vi "add channel.vi"(6 "replace if found?(T)":bool, 8 "error in (no error)":errorcluster, 9 "DSFChannel info":T1, 10 "id":string, 11 "DSFConfiguration in":refnum<class "DSFConfiguration.lvclass">) -> (0 "error out":errorcluster, 1 "found?":bool, 3 "DSFConfiguration out":refnum<class "DSFConfiguration.lvclass">)   [LabVIEW 2017, in "DSFConfiguration.lvclass"]
uses:
  DSFConfiguration.lvclass
  DSFConfiguration.lvclass/DSFConfiguration.ctl
  DSFChannel/DSFChannel.lvclass
  <vilib>/Utility/error.llb/Error Cluster From Error Code.vi
  <vilib>/ErrorRing/Error Ring.xnode
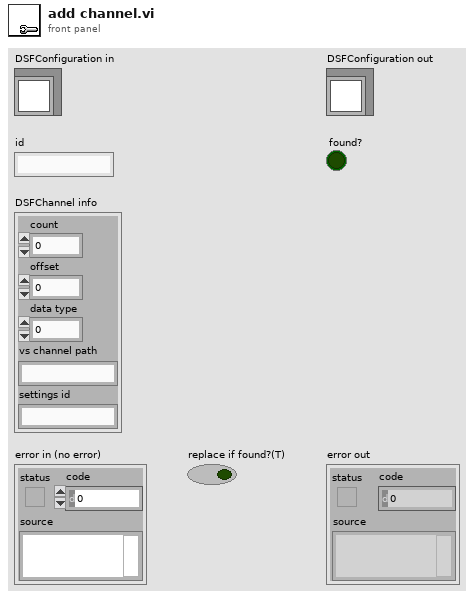
[diagram p1: front panel]
types:
  T1 = cluster{"count":i32, "offset":i32, "data type":i32, "vs channel path":string, "settings id":string}
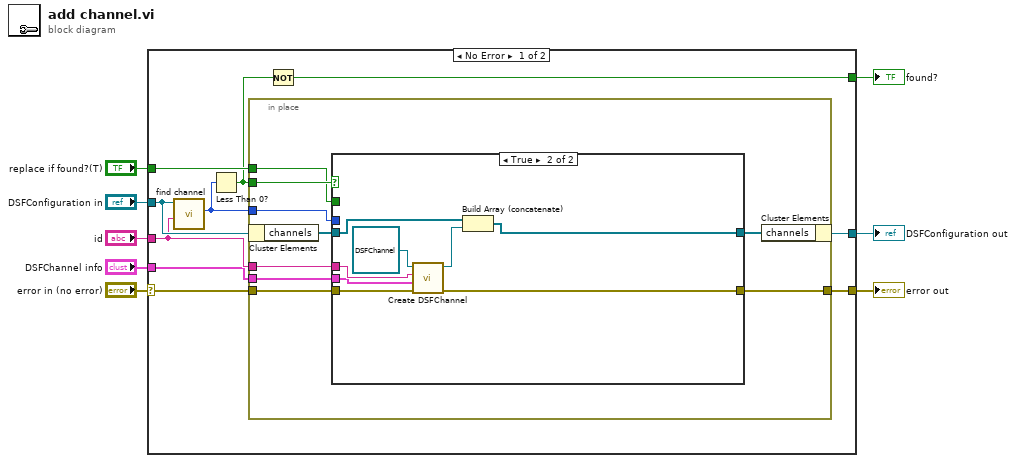
[diagram p0: block diagram]
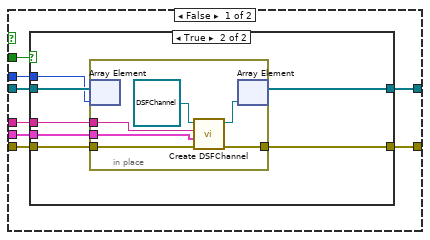
[diagram p2: hidden frame]
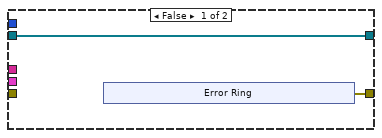
[diagram p3: hidden frame]
diagram:
  n1 = case shown="No Error" "error in (no error)" {
    selector: "error in (no error)" -> [w13 w64]
    tunnel: [w12 w64] -> w7
    tunnel: [w15 w63] -> w5
    tunnel: "DSFConfiguration in" -> [w18 w63]
    tunnel: "replace if found?(T)" -> [w17 _]
    tunnel: "id" -> [w14 _]
    tunnel: [w10 _] -> w2
    tunnel: "DSFChannel info" -> [w9 _]
    frame No Error {
      n2 = call "find channel.vi"("settings id"=w14, "DSFConfiguration in"=w18) -> ("index"=w16:i32)  [unwired: 9 in]
      n3 = Less Than 0?(x=w16) -> (x < 0?=w11:bool)
      n4 = in-place {
        in-place-border: w11 -> [w26]
        in-place-border: w14 -> [w25]
        in-place-border: w17 -> [w24]
        in-place-border: w16 -> [w23]
        in-place-border: w13 -> [w22]
        in-place-border: [w21] -> w12
        in-place-border: w9 -> [w20]
        n5 = in-place-cluster #1(w18) -> ("channels"=w27:refnum<class "DSFChannel.lvclass">[])
        n6 = case shown="True" w26 {
          tunnel: w27 -> [w35 w62]
          tunnel: w25 -> [w32 w59]
          tunnel: [w31 w61] -> w19
          tunnel: w24 -> [w34 _]
          tunnel: w23 -> [w33 _]
          tunnel: w22 -> [w30 w58]
          tunnel: [w29 w56] -> w21
          tunnel: w20 -> [w28 w55]
          frame False {
            n7 = case shown="True" w34 {
              tunnel: w35 -> [w37 w48]
              tunnel: w33 -> [_ w47]
              tunnel: w32 -> [_ w46]
              tunnel: [w37 w45] -> w31
              tunnel: w30 -> [_ w44]
              tunnel: [w36 w43] -> w29
              tunnel: w28 -> [_ w42]
              frame False {
                n8 = xnode "Error Ring"() -> ("error out"=w36:errorcluster)
              }
              frame True {
                n9 = in-place {
                  in-place-border: w46 -> [w53]
                  in-place-border: w44 -> [w51]
                  in-place-border: [w50] -> w43
                  in-place-border: w42 -> [w49]
                  n10 = in-place-array #2(w48, w47) -> ()  [unwired: 1 out]
                  n11 = call "Create DSFChannel.vi"("error in (no error)"=w51, "DSFChannel info"=w49, "id"=w53, "DSFChannel in"=refnum<class "DSFChannel.lvclass"> refnum ("DSFPluginSettings in")) -> ("error out"=w50:errorcluster, "DSFChannel out"=w52:refnum<class "DSFChannel.lvclass">)  [unwired: 6 in]
                  n12 = in-place-array #2(w52) -> (w45:refnum<class "DSFChannel.lvclass">[])  [unwired: 1 out]
                }
              }
            }
          }
          frame True {
            n13 = call "Create DSFChannel.vi"("error in (no error)"=w58, "DSFChannel info"=w55, "id"=w59, "DSFChannel in"=refnum<class "DSFChannel.lvclass"> refnum ("DSFPluginSettings in")) -> ("error out"=w56:errorcluster, "DSFChannel out"=w57:refnum<class "DSFChannel.lvclass">)  [unwired: 6 in]
            n14 = Build Array (concatenate)(w62, w57) -> (w61:refnum<class "DSFChannel.lvclass">[])
          }
        }
        n15 = in-place-cluster #1("channels"=w19) -> (w15:refnum<class "DSFConfiguration.lvclass">)
      }
      n16 = Not(x=w11) -> (.not. x?=w10:bool)
    }
    frame Error {
    }
  }
  "error out" <- w7
  "DSFConfiguration out" <- w5
  "found?" <- w2
